vi "onCreate.vi"(8 "error in (no error)":errorcluster, 11 "System":refnum<class "System.lvclass">) -> (0 "error out":errorcluster, 3 "System out":refnum<class "System.lvclass">)   [LabVIEW 2014, in "System.lvclass"]
doc: "JKI State Machine Objects (SMO) 1.4.0.57\nJKI - JKI\nCopyright (c) 2018, JKI"
uses:
  System.lvclass
  Query Payload -- cluster.ctl
  System.lvclass/System.ctl
  <vilib>/JKI/JKI SMO/SMO/SMO.lvclass
panel:
  # "For instructions on how to use the JKI State Machine Objects, examples and video tutorials, visit:\nhttp://jki.net/state-machine-objects/\n\nJKI State Machine Objects™\nhttp://jki.net/state-machine-objects/\nCopyright (C) 2005-2015, JKI <info@jki.net>\nALL RIGHTS RESERVED"
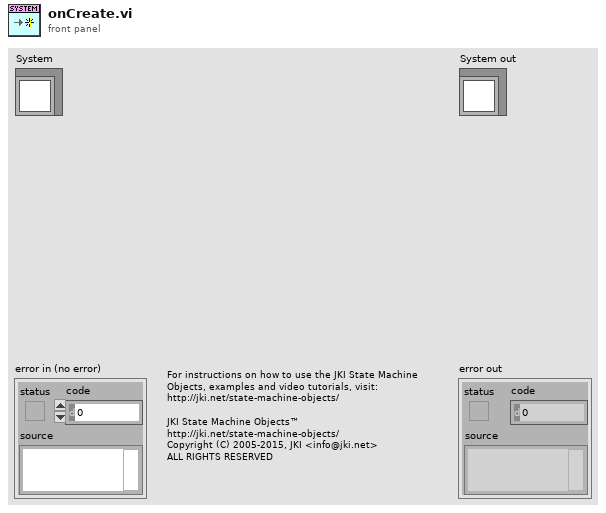
[diagram p1: front panel]
types:
  T1 = typedef "System.lvclass/Query Payload -- cluster.ctl" = cluster{"setpoint":dbl, "notifier":refnum<notifier>}
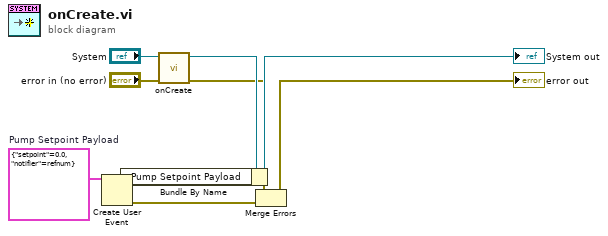
[diagram p0: block diagram]
diagram:
  w3 = T1 {"setpoint"=0.0, "notifier"=refnum}  # Pump Setpoint Payload
  n1 = Create User Event(user event datatype=w3) -> (user event=w2:refnum<user-event>, error out=w1:errorcluster)  [unwired: 1 in]
  n2 = call-parent "onCreate.vi"("error in (no error)"="error in (no error)", "SMO"="System") -> ("error out"=w5:errorcluster, "SMO out"=w9:refnum<class "System.lvclass">)  [unwired: 8 in]
  n3 = Bundle By Name(cluster=w9, "Pump Setpoint Payload"=w2) -> (→"System out":refnum<class "System.lvclass">)
  n4 = Merge Errors(w5, w1) -> (→"error out":errorcluster)
